vi "Stop Core.vi"(10 "final error code":i32, 11 "Controller in":refnum<class "Controller.lvclass">) -> (3 "Controller out":refnum<class "Controller.lvclass">)   [LabVIEW 2017, in "Controller Actor.lvlib" / "Controller.lvclass"]
uses:
  Controller.lvclass
  Controller.lvclass/Controller.ctl
  <vilib>/ActorFramework/Message Enqueuer/Message Enqueuer.lvclass/Message Enqueuer.ctl
  <vilib>/ActorFramework/Message Enqueuer/Enqueue.vi
  <vilib>/ActorFramework/Stop Msg/Stop Msg.lvclass
  C:/Program Files (x86)/National Instruments/LabVIEW 2017/vi.lib/ActorFramework/Message/Message.lvclass
  User Interface/Messages/Disable UI Msg/Disable UI Msg.lvclass
  <vilib>/ActorFramework/Message Priority Queue/Priority Enqueue.vi
  <vilib>/ActorFramework/Message Enqueuer/Message Enqueuer.lvclass
  <vilib>/ActorFramework/Actor/Actor.lvclass
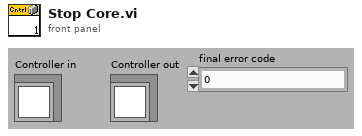
[diagram p1: front panel]
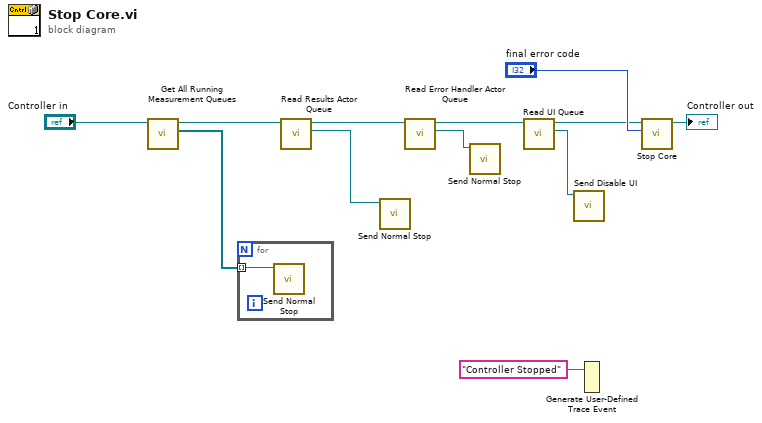
[diagram p0: block diagram]
diagram:
  n1 = call "Get All Running Measurement Queues.vi"("Controller in"="Controller in") -> ("Array of Measurement Queues"=w11:refnum<class "Message Enqueuer.lvclass">[], "Controller out"=w10:refnum<class "Controller.lvclass">)  [unwired: 8 in, 1 out]
  n2 = for {
    tunnel: w11 -> [w13] mode=indexing
    n3 = call <vilib>:"Send Normal Stop.vi"("Message Enqueuer"=w13) -> ()  [unwired: 10 in, 1 out]
  }
  n4 = call "Read Results Actor Queue.vi"("Controller in"=w10) -> ("Message Enqueuer"=w8:refnum<class "Message Enqueuer.lvclass">, "Controller out"=w6:refnum<class "Controller.lvclass">)  [unwired: 8 in, 1 out]
  n5 = call <vilib>:"Send Normal Stop.vi"("Message Enqueuer"=w8) -> ()  [unwired: 10 in, 1 out]
  n6 = call "Read Error Handler Actor Queue.vi"("Controller in"=w6) -> ("Actor Framework.lvlib:Message Enqueuer"=w5:refnum<class "Message Enqueuer.lvclass">, "Controller out"=w3:refnum<class "Controller.lvclass">)  [unwired: 8 in, 1 out]
  n7 = call <vilib>:"Send Normal Stop.vi"("Message Enqueuer"=w5) -> ()  [unwired: 10 in, 1 out]
  n8 = call "Read UI Queue.vi"("UI Controller in"=w3) -> ("UI Queue"=w1:refnum<class "Message Enqueuer.lvclass">, "UI Controller out"=w2:refnum<class "Controller.lvclass">)  [unwired: 8 in, 1 out]
  n9 = call "Send Disable UI.vi"("Message Enqueuer"=w1) -> ()  [unwired: 9 in, 2 out]
  n10 = Generate User-Defined Trace Event(2:"Controller Stopped" ("trace string")) -> ()  [unwired: 1 in]
  n11 = call-parent "Stop Core.vi"("final error code"="final error code", "Actor in"=w2) -> ("Actor out"=→"Controller out":refnum<class "Controller.lvclass">)  [unwired: 9 in]
